vi "FTW-CodeGen-GenerateCode.vi"(0 "State In":T2, 5 "XRef":refnum<vi>, 7 "Terms":T1(array[cluster]), 9 "Diagram":refnum<vi>) -> (4 "State Out":T2, 6 "Reply":string[](array[string]), 8 "Generated Code?":bool)   [LabVIEW 2014, in "FTW-Array-Shuffle.xnode"]
uses:
  FTW-Array-Shuffle.xnode
  FTW-CodeGen-State.ctl
  FTW-CodeGen-XNodeReplyType.ctl
panel:
  # "Inputs"
  # "Outputs"
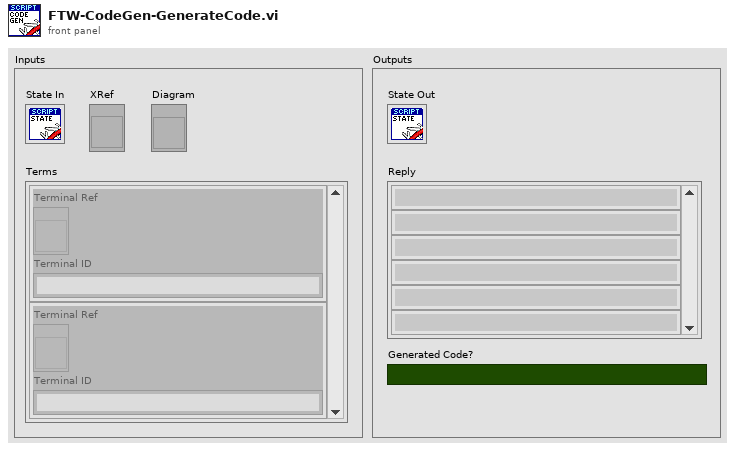
[diagram p1: front panel]
types:
  T1 = cluster{"Terminal Ref":refnum<vi>, "Terminal ID":string}[]
  T2 = typedef "FTW-Array-Shuffle.xnode/FTW-CodeGen-State.ctl" = cluster{"Dummy":string}
  T3 = typedef "FTW-CodeGen-XNodeReplyType.ctl" = enum16{"UpdateState", "AdaptToInputs", "AdaptAndAugment", "CosmeticUpdate", "NoReply"}
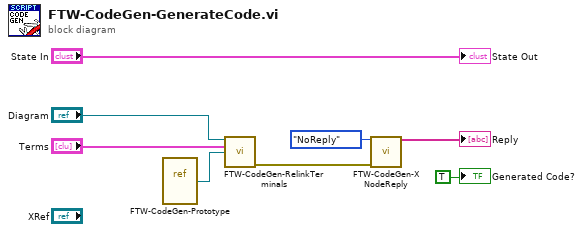
[diagram p0: block diagram]
diagram:
  n1 = vi-ref "FTW-CodeGen-Prototype.vi"() -> (w2:refnum<vi>)
  n2 = call "FTW-CodeGen-RelinkTerminals.vi"("Diagram"="Diagram", "Terms"="Terms", "PrototypeVI"=w2) -> ("error out"=w5:errorcluster)  [unwired: 11 in, 1 out]
  n3 = call "FTW-CodeGen-XNodeReply.vi"("XNode Reply Type"=FTW-CodeGen-XNodeReplyType."NoReply", "error in"=w5) -> ("Reply"=→"Reply":string[])  [unwired: 13 in]
  "State Out" <- "State In"
  "Generated Code?" <- TRUE ("Generated Code?")
